vi "SimulatedFGV.vi"(10 "Starting Temperature":dbl, 11 "FGV Function":T1=enum."Set On") -> (3 "Current Temperature":dbl=0.1)   [LabVIEW 2013]
uses:
  Controls/FGV Function.ctl
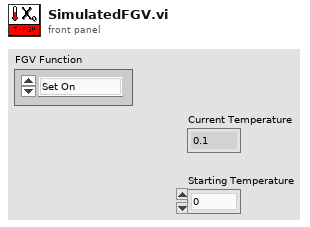
[diagram p1: front panel]
types:
  T1 = typedef "FGV Function.ctl" = enum16{"Initiate", "Read", "Set On", "Set Off"}
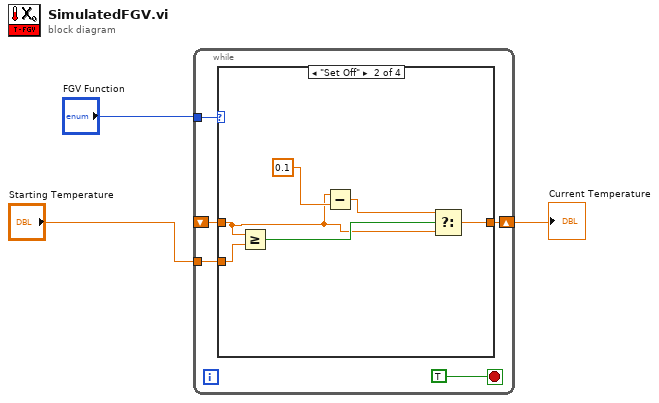
[diagram p0: block diagram]
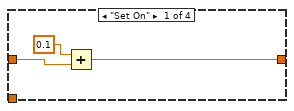
[diagram p2: hidden frame]
diagram:
  n1 = while {
    shift-right: [w6] -> w2
    shift-left: _ -> [w5]
    tunnel: "FGV Function" -> [w7]
    tunnel: "Starting Temperature" -> [w4]
    stop <- TRUE stop-if-true
    n2 = case shown="\"Set Off\"" w7 {
      tunnel: [w9 w15 w18 w19] -> w6
      tunnel: w5 -> [w11 w12 w18 _]
      tunnel: w4 -> [_ w17 _ w19]
      frame "Set On" {
        n3 = Add(x=0.1, y=w11) -> (x+y=w9:dbl)
      }
      frame "Set Off" {
        n4 = Greater Or Equal?(x=w12, y=w17) -> (x >= y?=w16:bool)
        n5 = Subtract(x=w12, y=0.1 ("x")) -> (x-y=w14:dbl)
        n6 = Select(t=w14, s=w16, f=w12) -> (s? t:f=w15:dbl)
      }
      frame "Read" {
      }
      frame "Initiate" {
      }
    }
  }
  "Current Temperature" <- w2
